vi "Error - Log.vi"(8 "error in (no error)":errorcluster, 11 "Error Event":T1) -> (0 "error out":errorcluster)   [LabVIEW 2017]
doc: "This SubVI serves for maintains a log file with error handling information.\n[Covers: EH4]"
uses:
  Controls/Error Event.ctl
  Controls/Error Type.ctl
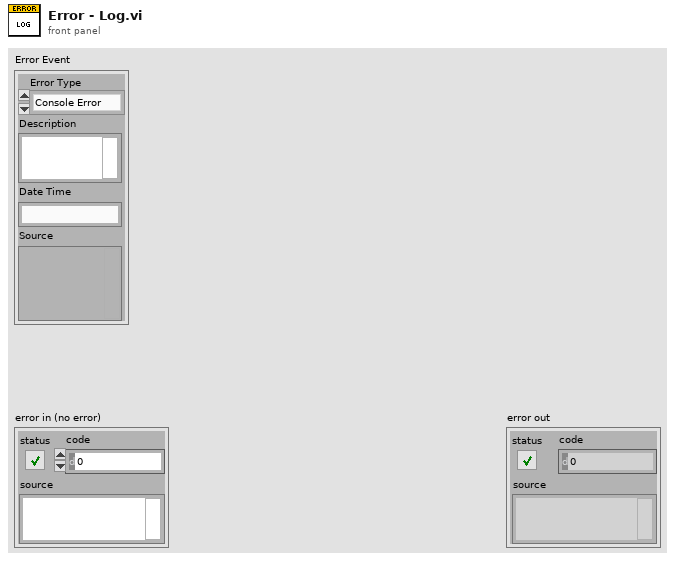
[diagram p1: front panel]
types:
  T1 = typedef "Error Event.ctl" = cluster{"Error Type":T2, "Description":string, "Date Time":string, "Source":variant}
  T2 = typedef "Error Type.ctl" = enum16{"Console Error", "Sensor Interface IO Error", "Process Step Error"}
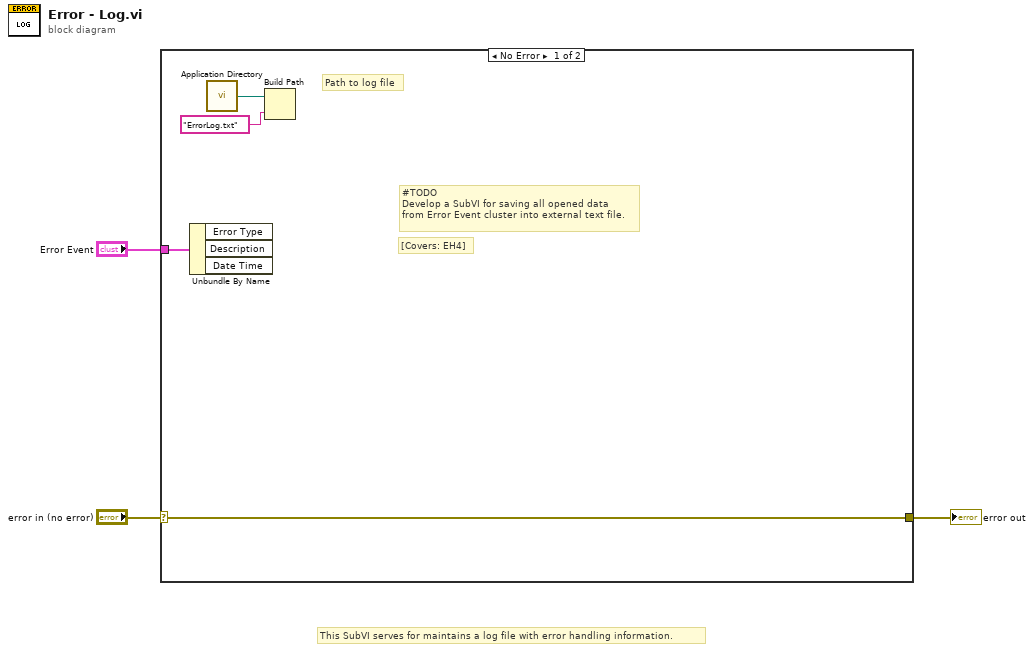
[diagram p0: block diagram]
diagram:
  # "This SubVI serves for maintains a log file with error handling information."
  n1 = case shown="No Error" "error in (no error)" {
    selector: "error in (no error)" -> [w7 w8]
    tunnel: [w7 w8] -> w2
    tunnel: "Error Event" -> [w4 _]
    frame No Error {
      # "[Covers: EH4]"
      # "Path to log file"
      # "#TODO\nDevelop a SubVI for saving all opened data\nfrom Error Event cluster into external text file."
      n2 = Unbundle By Name(w4) -> ()  [unwired: 3 out]
      n3 = call <vilib>:"Application Directory.vi"() -> ("Application Directory"=w6:path)
      n4 = Build Path(base path=w6, name or relative path="ErrorLog.txt") -> ()  [unwired: 1 out]
    }
    frame Error {
    }
  }
  "error out" <- w2
